vi "Simple Reader.vi"(8 "error in (no error)":errorcluster, 11 "rotator driver in":refnum<class "rotator driver.lvclass">) -> (0 "error out":errorcluster, 2 "Signals":dbl[](array[numeric]), 3 "rotator driver out":refnum<class "rotator driver.lvclass">)   [LabVIEW 2018, in "rotator driver.lvclass"]
uses:
  rotator driver.lvclass
  stepper driver action.ctl
  stepper driver -- BLM.vi
  stepper driver -- IMS.vi
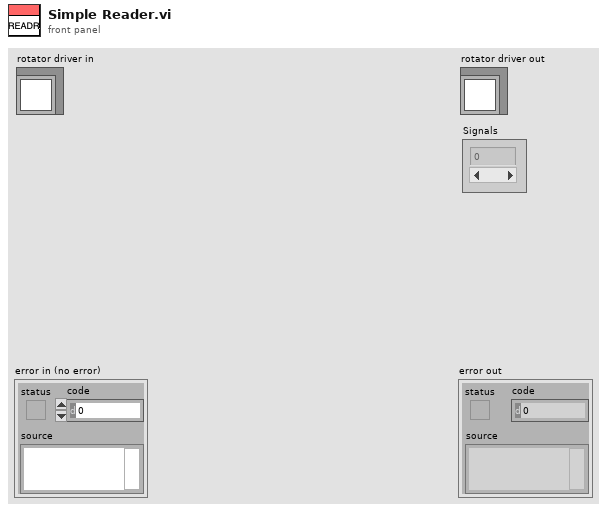
[diagram p1: front panel]
types:
  T1 = typedef "stepper driver action.ctl" = enum16{"go", "void", "stop", "check", "init", "sync", "set", "set speed", "--check status", "--check value"}
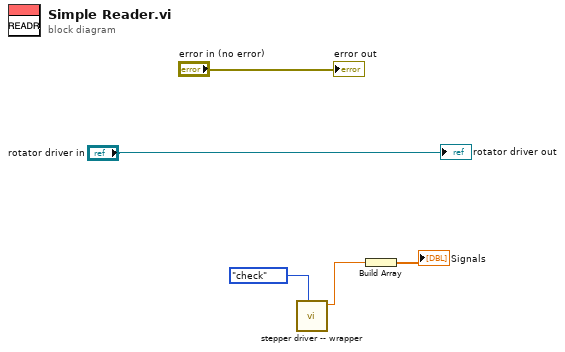
[diagram p0: block diagram]
diagram:
  n1 = call "stepper driver -- wrapper.vi"("stepper driver action"=stepper_driver_action."check") -> ("number OUT"=w2:dbl)  [unwired: 8 in, 2 out]
  n2 = Build Array(w2) -> (→"Signals":dbl[])
  "error out" <- "error in (no error)"
  "rotator driver out" <- "rotator driver in"
